vi "FERRICCH.vi"() -> ()   [LabVIEW 2016]
doc: "This example performs writes and reads on a serial port, as directed by the user. You can press the Write and Read buttons, and change the Read Count, while the example is running.\n\nThe parameters set for the serial port must match the parameters of the connected instrument or device. In this example, the Read Count parameter specifies the number of bytes that the serial port reads. If there were more bytes at the port than the specified number, those bytes would not be read. If there were less bytes at the port than the specified number, you would receive a timeout error.\n\nThis example expands upon the flow control options for XON and XOFF, allowing the user to choose those control characters. Also, the user can enable or disable a termination character. Some devices require a termination character in order to identify the end of command strings. Some devices send a termination character to signify the end of data to be read. This example shows how you can end the Read operation once a termination character is detected in the buffer and/or append a termination character at the end of the Write data."
uses:
  Program Files/National Instruments/LabVIEW 2016/examples/Instrument IO/Serial/support/Serial - Settings.ctl
  Program Files/National Instruments/LabVIEW 2016/examples/Instrument IO/Serial/support/Serial - XON-XOFF Characters.ctl
  Program Files/National Instruments/LabVIEW 2016/examples/Instrument IO/Serial/support/Serial - ASCII Characters.ctl
  <vilib>/Instr/_visa.llb/VISA Configure Serial Port (Instr).vi
  <vilib>/express/express arith-compare/Formula/XNode/ExpressFormulaBlockNode.xnode
panel:
  out "Waveform Chart":dbl[](graph)
  in  "Save File?":bool
  in  "Lower Limit":dbl
  in  "Upper Limit":dbl
  out "Time of Program":dbl
  out "Program End Time":dbl
  out "Concentration M (moldm-3)":string
  in  "Write":bool
  in  "Start Read":bool
  in  "No of Data":i32
  in  "Time per Data":i32
  in  "Serial Settings":T1={"baud rate"=9600, "data bits"=8, "parity"=enum."None", "stop bits"=10, "flow control"=0} {"flow control" items=["None"=0, "XON/XOFF"=1, "RTS/CTS"=2, "DTR/DSR"=4]; "stop bits" items=["1.0"=10, "1.5"=15, "2.0"=20]; "data bits" min=5 max=8 step=1; "baud rate" items=["75"=75, "110"=110, "134"=134, "150"=150, "300"=300, "600"=600, "1200"=1200, "1800"=1800, "2400"=2400, "4800"=4800, "7200"=7200, "9600"=9600, "14400"=14400, "19200"=19200, "28800"=28800, "38400"=38400, "56000"=56000, "57600"=57600, "115200"=115200, "128000"=128000, "230400"=230400]}
  in  "Command":string="*IDN?"
  in  "Termination Character":u8=10 format="%.0x"
  in  "VISA resource name":refnum<visa-resource-name>="COM1"
  in  "Read Count":u32=1000
  in  "XON/XOFF Characters":T2={"XON"=enum."DC1", "XOFF"=enum."DC3"}
  out "Concentration LOW":bool
  out "Concentration High":bool
  in  "?":bool=TRUE
  in  "?":bool=TRUE
  # "endd"
  # "aad"
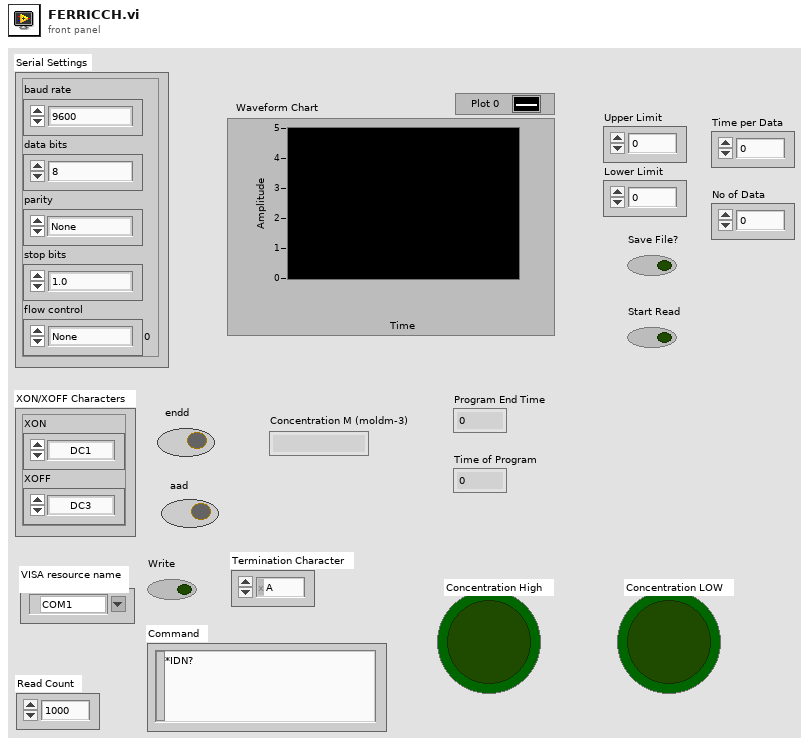
[diagram p1: front panel]
types:
  T1 = typedef "Serial - Settings.ctl" = cluster{"baud rate":u32, "data bits":u16, "parity":enum16{"None", "Odd", "Even", "Mark", "Space"}, "stop bits":u16, "flow control":u16}
  T2 = typedef "Serial - XON-XOFF Characters.ctl" = cluster{"XON":T3, "XOFF":T3}
  T3 = typedef "Serial - ASCII Characters.ctl" = enum16{"NUL", "SOH", "STX", "ETX", "EOT", "ENQ", "ACK", "BEL", "BS", "HT", "LF", "VT", "FF", "CR", "SO", "SI", "DLE", "DC1", "DC2", "DC3", "DC4", "NAK", "SYN", "ETB", "CAN", "EM", "SUB", "ESC", "FS", "GS", "RS", "US", "SP", "!", "\"", "#", "$", "%", "&", "'", "(", ")", "*", "+", ",", "- (-)", ".", "/", "0", "1", "2", "3", "4", "5", "6", "7", "8", "9", ":", ";", "<", "=", ">", "?", "@", "A", "B", "C", "D", "E", "F", "G", "H", "I", "J", "K", "L", "M", "N", "O", "P", "Q", "R", "S", "T", "U", "V", "W", "X", "Y", "Z", "[", "\\", "]", "^", "_", "`", "a", "b", "c", "d", "e", "f", "g", "h", "i", "j", "k", "l", "m", "n", "o", "p", "q", "r", "s", "t", "u", "v", "w", "x", "y", "z", "{", "|", "}", "~"}
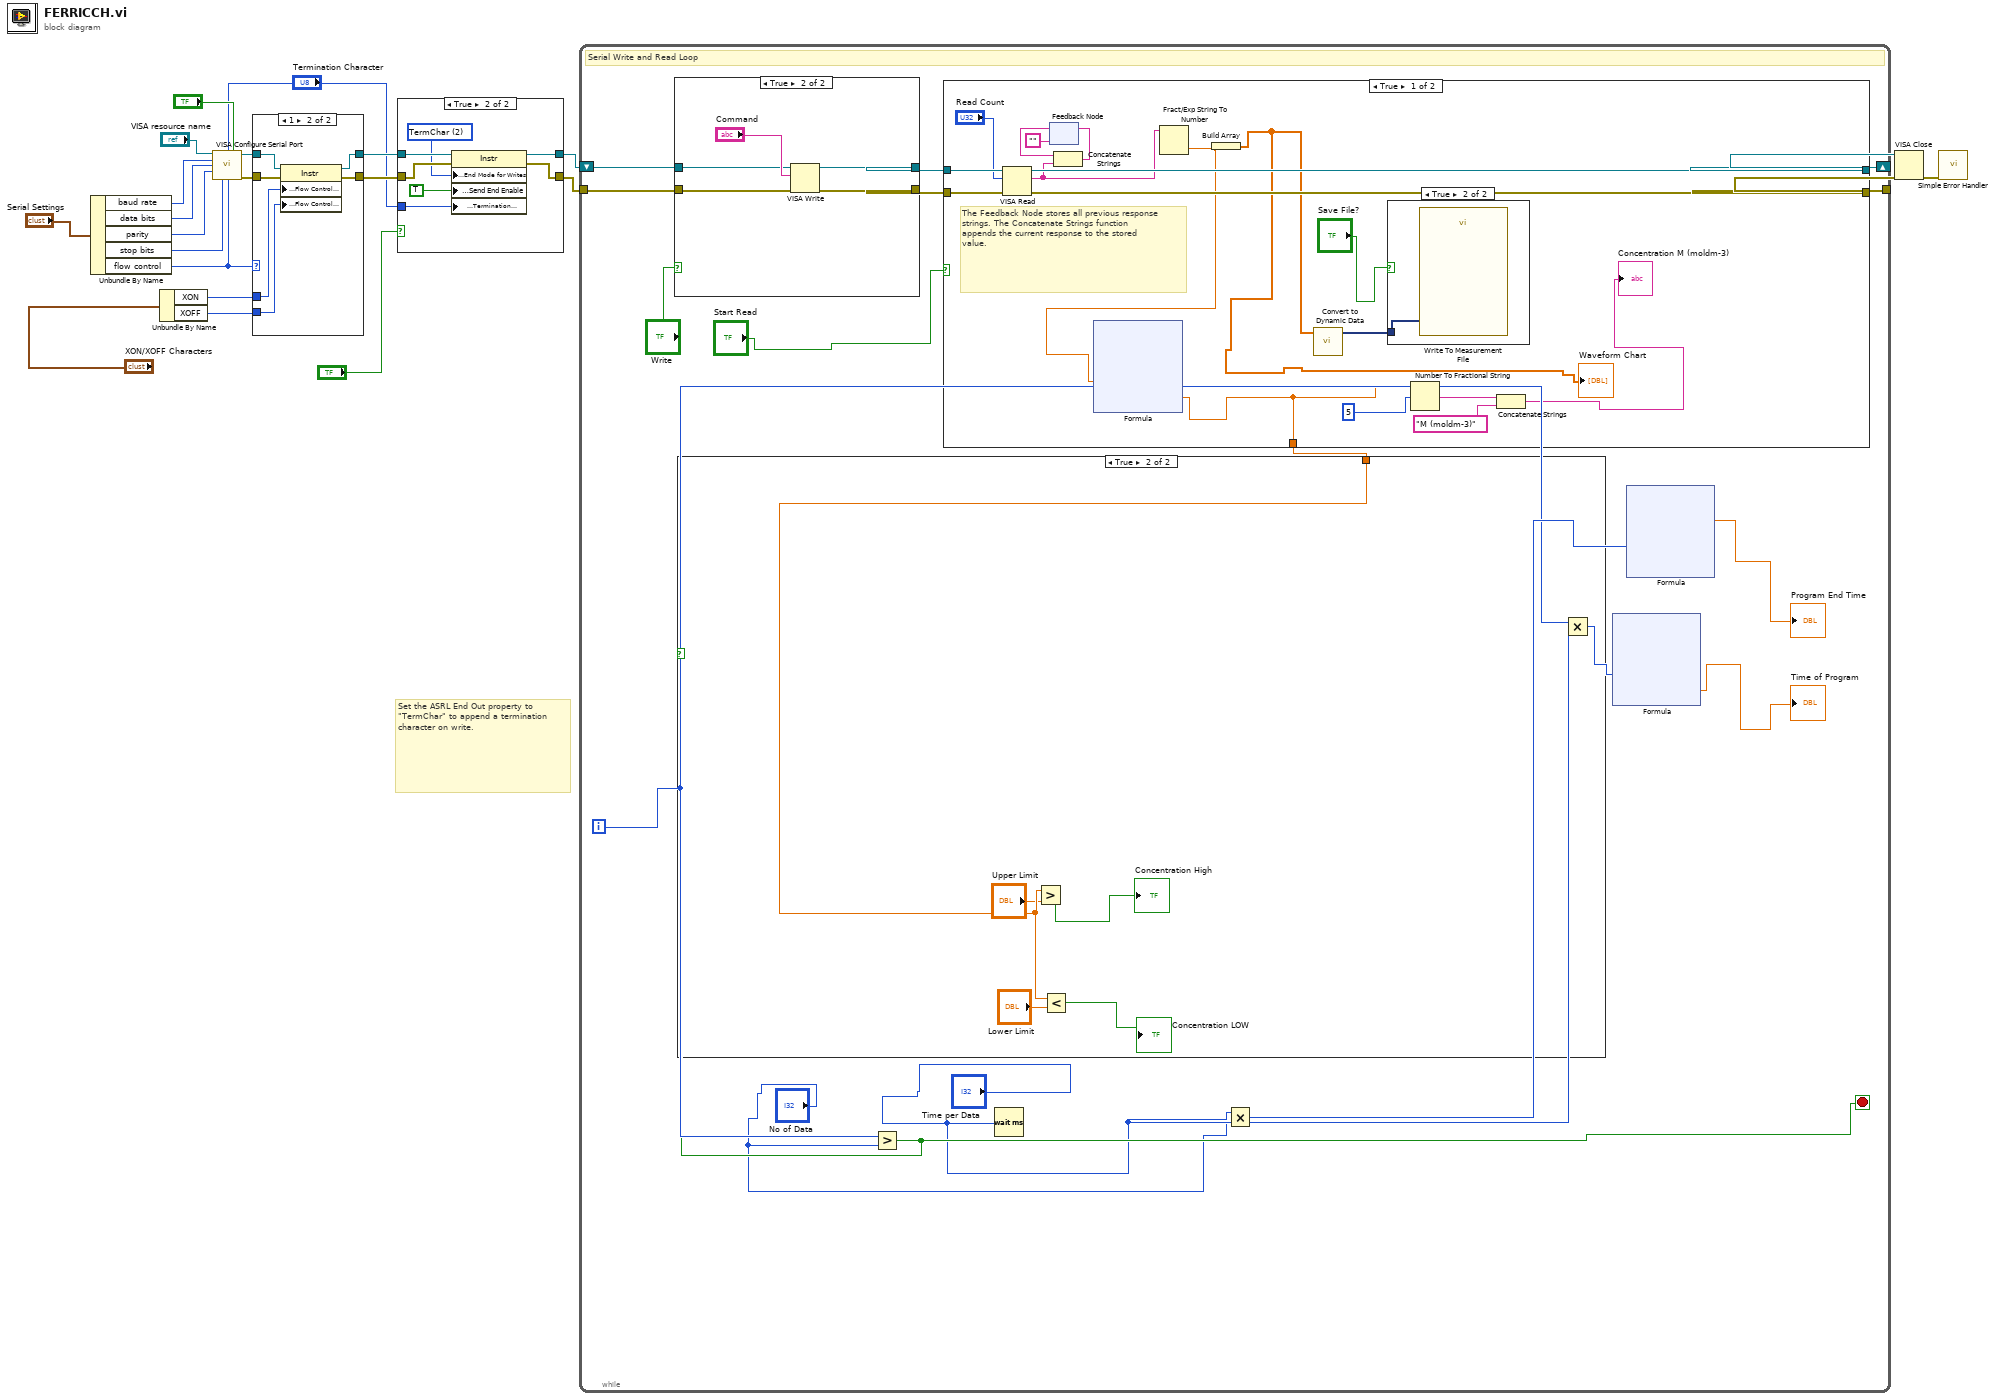
[diagram p0: block diagram]
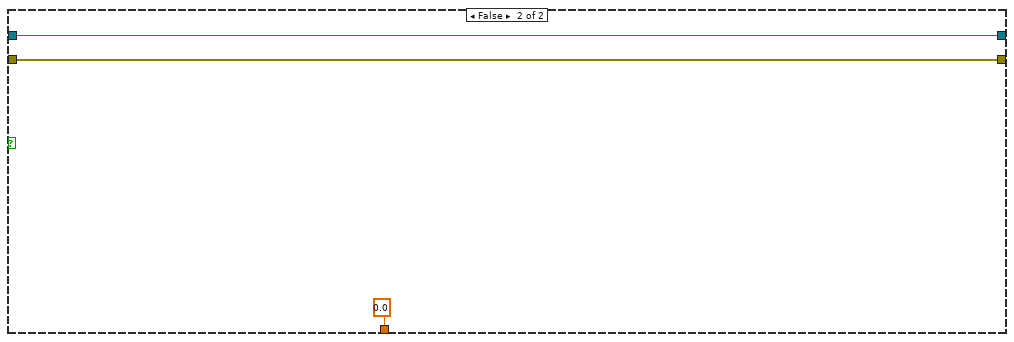
[diagram p7: hidden frame]
diagram:
  # "Set the ASRL End Out property to \"TermChar\" to append a termination character on write."
  n1 = Unbundle By Name("Serial Settings") -> ("baud rate"=w15:u32, "data bits"=w16:u16, "parity"=w17:enum16{"None", "Odd", "Even", "Mark", "Space"}, "stop bits"=w18:u16, "flow control"=w9:u16)
  n2 = Unbundle By Name("XON/XOFF Characters") -> ("XON"=w8:T3, "XOFF"=w7:T3)
  n3 = call-poly "VISA Configure Serial Port"("VISA resource name"="VISA resource name", "termination char\n(0xA = '\\n' = LF)"="Termination Character", "Enable Termination\nChar (T)"="?", "baud rate (9600)"=w15, "data bits (8)"=w16, "parity (0:none)"=w17, "stop bits (10: 1 bit)"=w18, "flow control (0:none)"=w9) -> ("VISA resource name out"=w19:refnum<visa-resource-name>, "error out"=w20:errorcluster)  [unwired: 2 in, 4 out]
  n4 = case shown="1" w9 {
    tunnel: [w23 w30] -> w6
    tunnel: [w24 w29] -> w4
    tunnel: w20 -> [w23 w28]
    tunnel: w19 -> [w24 w27]
    tunnel: w8 -> [_ w26]
    tunnel: w7 -> [_ w25]
    frame Default {
    }
    frame 1 {
      n5 = property class="Instr"(reference=w27, error in=w28, "Serial Settings:Flow Control XON Character"=w26, "Serial Settings:Flow Control XOFF Character"=w25) -> (reference out=w29:refnum<visa-resource-name>, error out=w30:errorcluster)
    }
  }
  n6 = case shown="True" "?" {
    tunnel: w4 -> [w31 w39]
    tunnel: w6 -> [w32 w38]
    tunnel: [w31 w37] -> w3
    tunnel: [w32 w36] -> w5
    tunnel: "Termination Character" -> [_ w34]
    frame False {
    }
    frame True {
      w35 = u16 2 items=["None", "LastBit", "TermChar", "Break"] ("Serial Settings:Serial End Mode for Writes")
      n7 = property class="Instr"(reference=w39, error in=w38, "Serial Settings:End Mode for Writes"=w35, "Message Based Settings:Send End Enable"=TRUE, "Message Based Settings:Termination Character"=w34) -> (reference out=w37:refnum<visa-resource-name>, error out=w36:errorcluster)
    }
  }
  n8 = while {
    shift-right: [w56] -> w10
    shift-left: w3 -> [w55]
    tunnel: w5 -> [w54]
    tunnel: [w51] -> w11
    i -> [w48]
    stop <- w47 stop-if-true
    # "Serial Write and Read Loop"
    n9 = case shown="True" "Write" {
      tunnel: w55 -> [w79 w83]
      tunnel: w54 -> [w78 w82]
      tunnel: [w79 w81] -> w53
      tunnel: [w78 w80] -> w52
      frame False {
      }
      frame True {
        n10 = VISA Write(VISA resource name=w83, write buffer="Command", error in (no error)=w82) -> (VISA resource name out=w81:refnum<visa-resource-name>, error out=w80:errorcluster)  [unwired: 1 out]
      }
    }
    n11 = Greater?(x=w48, y="No of Data") -> (0:w47:bool)
    n12 = case shown="True" "Start Read" {
      tunnel: [w100 w114] -> w56
      tunnel: w53 -> [w102 w114]
      tunnel: [w98 w113] -> w51
      tunnel: w52 -> [w101 w113]
      tunnel: [w88 0.0 ("Result")] -> w46
      frame True {
        # "The Feedback Node stores all previous response strings. The Concatenate Strings function appends the current response to the stored value."
        n13 = VISA Read(VISA resource name=w102, byte count="Read Count", error in (no error)=w101) -> (VISA resource name out=w100:refnum<visa-resource-name>, read buffer=w94:string, error out=w98:errorcluster)  [unwired: 1 out]
        n14 = feedback #1("") -> (w97:string)
        n15 = Concatenate Strings(w97, w94) -> (w95:string)
        n16 = feedback-in #1(w95) -> ()
        n17 = Fract/Exp String To Number(string=w94) -> (number=w92:dbl)  [unwired: 3 in, 1 out]
        n18 = xnode "Formula"("X1"=w92) -> ("Result"=w88:dbl)  [unwired: 1 in, 1 out]
        n19 = Build Array(w92) -> (w85:dbl[])
        "Waveform Chart" <- w85
        n20 = call "Convert to Dynamic Data"("Array"=w85) -> ("Dynamic Data Type"=w93:dynamicdata)  [unwired: 3 in]
        n21 = case shown="True" "Save File?" {
          tunnel: w93 -> [_ w111]
          frame False {
          }
          frame True {
            n22 = call "Write To Measurement File"("Signals"=w111) -> ()  [unwired: 16 in, 3 out]
          }
        }
        n23 = Number To Fractional String(number=w88, width (-)=i16 5) -> (F-format string=w90:string)  [unwired: 2 in]
        n24 = Concatenate Strings(w90, "M (moldm-3)" ("string")) -> (→"Concentration M (moldm-3)":string)
      }
      frame False {
      }
    }
    n25 = case shown="True" w47 {
      tunnel: w46 -> [_ w59]
      frame False {
      }
      frame True {
        n26 = Greater?(x=w59, y="Upper Limit") -> (0:→"Concentration High":bool)
        n27 = Less?(x=w59, y="Lower Limit") -> (x < y?=→"Concentration LOW":bool)
      }
    }
    n28 = Wait (ms)(milliseconds to wait="Time per Data") -> ()  [unwired: 1 out]
    n29 = Multiply(x="Time per Data", y="No of Data") -> (x*y=w50:i32)
    n30 = Multiply(x=w48, y="Time per Data") -> (x*y=w49:i32)
    n31 = xnode "Formula"("X1"=w49) -> ("Result"=→"Time of Program":dbl)  [unwired: 1 in, 1 out]
    n32 = xnode "Formula"("X1"=w50) -> ("Result"=→"Program End Time":dbl)  [unwired: 1 in, 1 out]
  }
  n33 = VISA Close(VISA resource name=w10, error in (no error)=w11) -> (error out=w12:errorcluster)
  n34 = call <vilib>:"Simple Error Handler.vi"("error in (no error)"=w12) -> ()  [unwired: 1 in, 8 out]
